vi "RRTAlgorithm2.vi"(0 "Dest x,y":dbl[](array[numeric]), 1 "Robot":T1={"id"=0, "function"=enum."Attacker", "x"=0.0, "y"=0.0, "orientation"=0.0, "v_tangent"=0.0, "v_normal"=0.0, "v_ang"=0.0, "kick_x"=0.0, "kick_z"=0.0, "dribble"=FALSE, "Timestamp"=timestamp(0 s since 1904-01-01), "estimatives"={"est_v_tangent"=0.0, "est_v_normal"=0.0, "est_vx"=0.0, "est_vy"=0.0, "Pos Robot Est"=[]}, "dest_x_kick"=0.0, "dest_y_kick"=0.0, "Gap Coord"=[], "States"=enum."Pass", "Path "=[], "Path  Smooth"=[], "Dest"=[], "vx_desired"=0.0, "vy_desired"=0.0, "slowBehavior"=FALSE, "VSSStates"=enum."Pass"}, 2 "WayPointProb":dbl, 3 "Path in \n(Smooth do Feedback Node)":dbl[][](array[numeric]), 4 "Step":dbl, 5 "GoalProb":dbl, 6 "Simple Path":dbl[][](array[numeric]), 7 "Ball":T7, 8 "Initial Pos x,y":dbl[](array[numeric]), 9 "our_robots":T1[](array[typedef]), 10 "Initial Pos 1,x,y,0":dbl[](array[numeric]), 11 "enemy_robots":T1[](array[typedef]), 12 "ignoreBall?":bool, 13 "Field Geomtery":u32[](array[numeric]), 19 "buffer":dbl[](array[numeric])) -> (16 "Path":dbl[][](array[numeric]))   [LabVIEW 2020]
uses:
  Vision_class/Old vision/SSL Detection Frame Simple Estimator Cameras VelCmd Folder/Core/AI Ball.ctl
  Vision_class/Old vision/Controls/AI Robot.ctl
  Vision_class/Old vision/Controls/Functions Enum.ctl
  Vision_class/Old vision/Controls/AttackerStates.ctl
  Vision_class/Old vision/Controls/PathDests.ctl
  Vision_class/Old vision/Controls/PathDest.ctl
  Navigation/VSSNavigation/VSSAttackerStates.ctl
  <vilib>/Analysis/_algsub.llb/Real Vector Norm.vi
  <vilib>/Analysis/coordinate.llb/2D Cartesian Coordinate Rotation (Scalar).vi
  <vilib>/Analysis/NI_AALPro.lvlib
panel:
  out "useSimplePath":i32
  out "pathsize":i32
  out "debug":sgl
  out "newTree":dbl[](array[numeric])
  in  "threshold":dbl=80.0
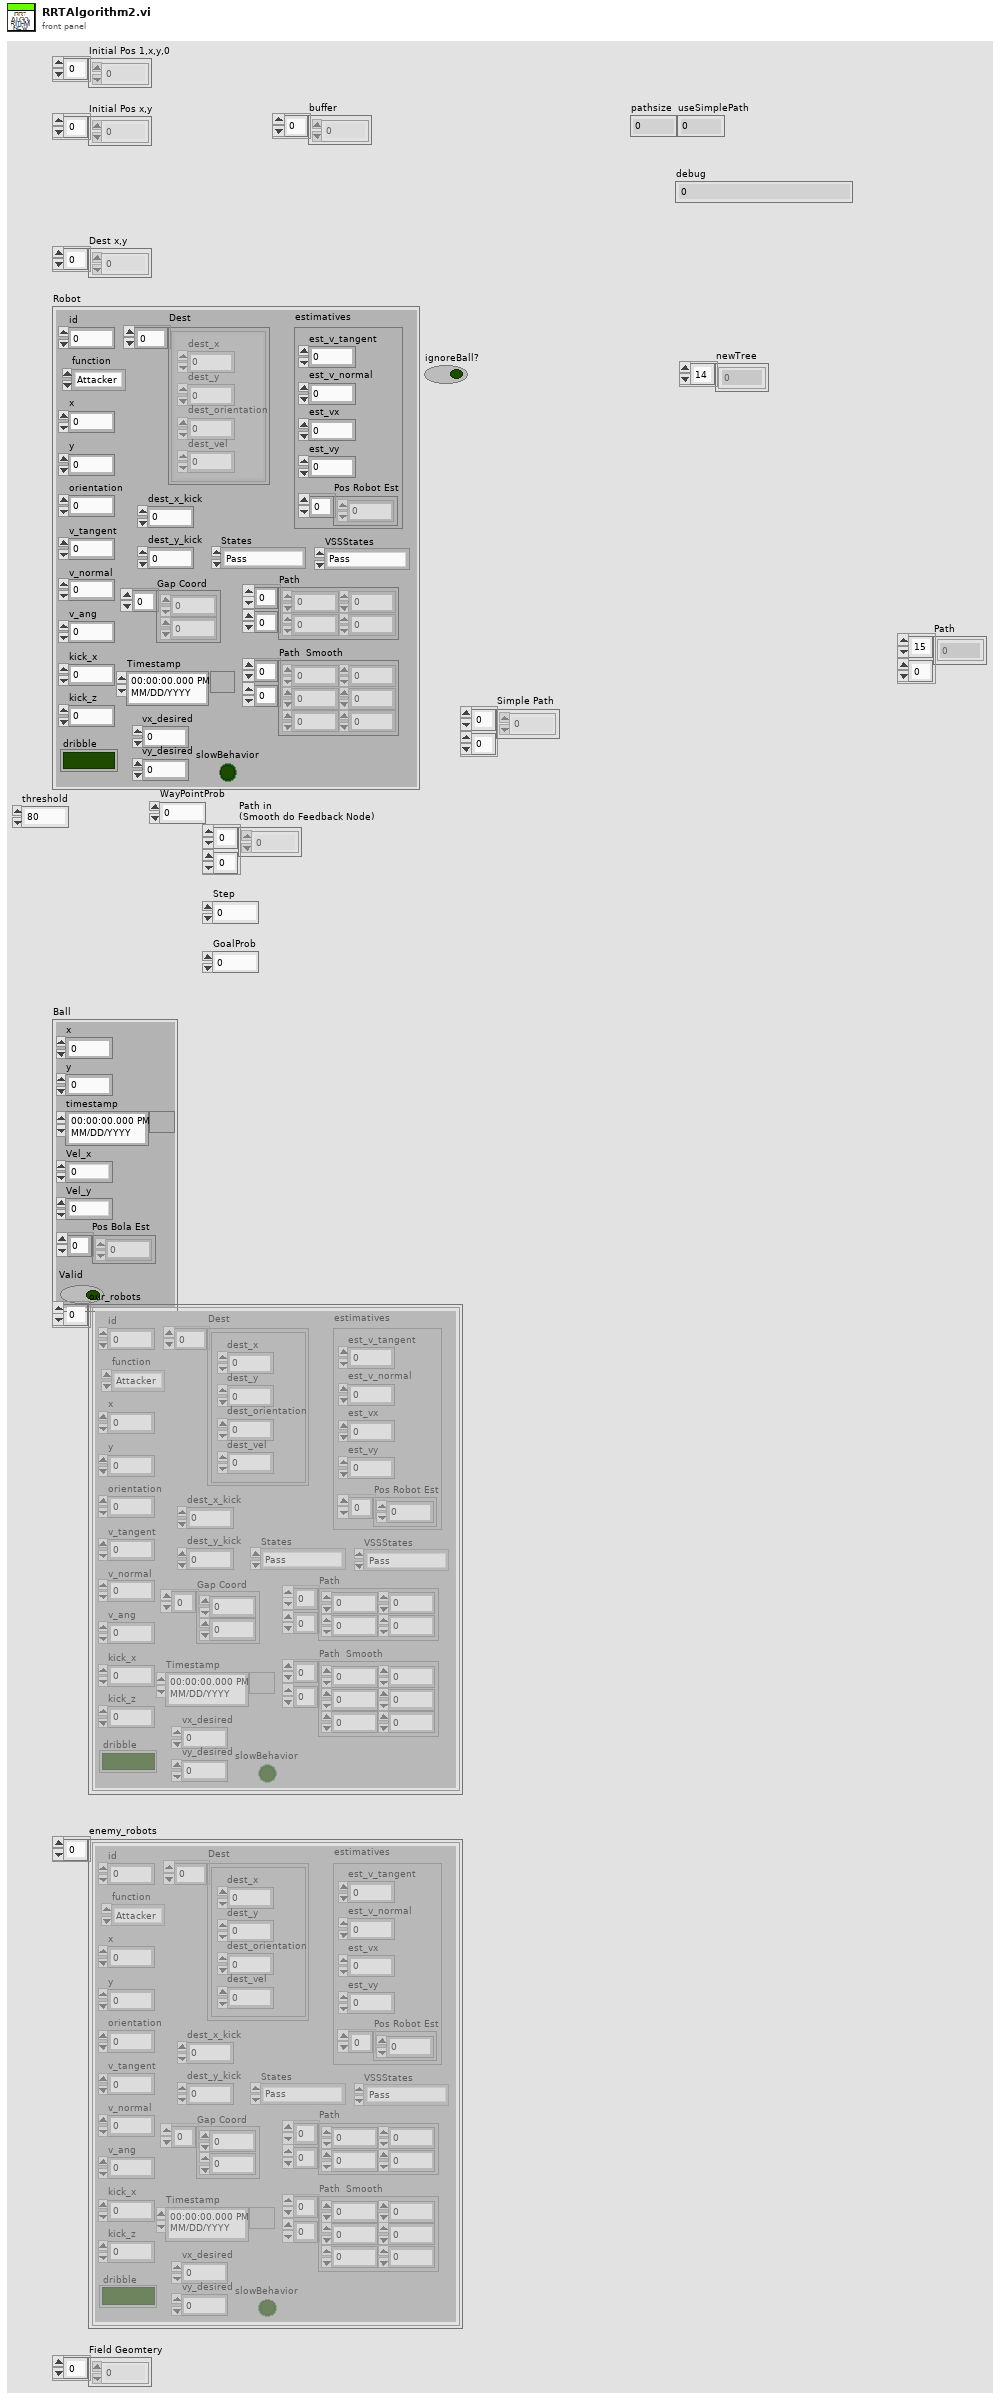
[diagram p1: front panel]
types:
  T1 = typedef "AI Robot.ctl" = cluster{"id":u32, "function":T2, "x":dbl, "y":dbl, "orientation":dbl, "v_tangent":dbl, "v_normal":dbl, "v_ang":dbl, "kick_x":dbl, "kick_z":dbl, "dribble":bool, "Timestamp":timestamp, "estimatives":cluster{"est_v_tangent":dbl, "est_v_normal":dbl, "est_vx":dbl, "est_vy":dbl, "Pos Robot Est":dbl[]}, "dest_x_kick":dbl, "dest_y_kick":dbl, "Gap Coord":dbl[], "States":T3, "Path ":dbl[][], "Path  Smooth":dbl[][], "Dest":T4, "vx_desired":dbl, "vy_desired":dbl, "slowBehavior":bool, "VSSStates":T6}
  T2 = typedef "Functions Enum.ctl" = enum16{"2nd Striker", "Attacker", "Goalie", "Defender", "Striker", "Goto 0", "Dummy", "Kicker", "ZigZag 0", "ZigZag 1", "ZigZag 2", "ZigZag 3", "ZigZag 4", "ZigZag 5", "ZigZag 6", "ZigZag 7", "ZigZag 8", ""}
  T3 = typedef "AttackerStates.ctl" = enum16{"Pass", "GoToTangent", "BallGetting", "GoToKick", ""}
  T4 = typedef "PathDests.ctl" = T5[]
  T5 = typedef "PathDest.ctl" = cluster{"dest_x":dbl, "dest_y":dbl, "dest_orientation":dbl, "dest_vel":dbl}
  T6 = typedef "VSSAttackerStates.ctl" = enum16{"Pass", "GoToTangent", "BallGetting", "GoToKick", "Rotate anti-clockwise", "Rotate Clockwise", ""}
  T7 = typedef "AI Ball.ctl" = cluster{"x":dbl, "y":dbl, "timestamp":timestamp, "Vel_x":dbl, "Vel_y":dbl, "Pos Bola Est":dbl[], "Valid":bool}
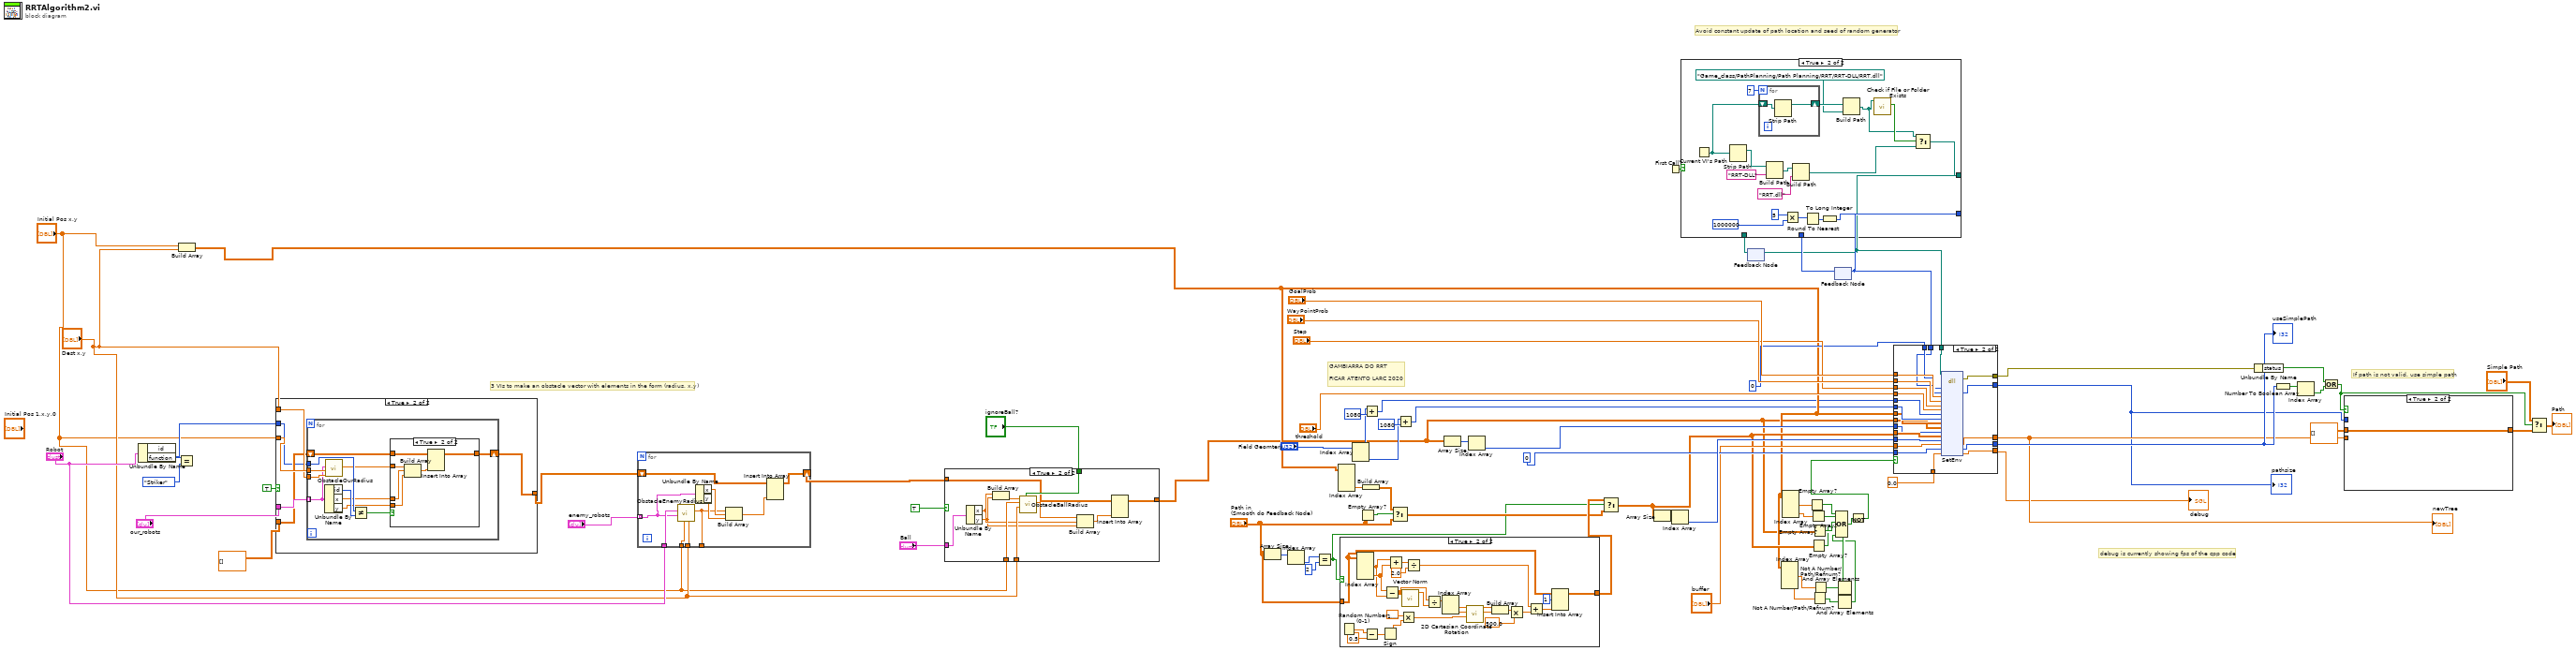
[diagram p0: block diagram]
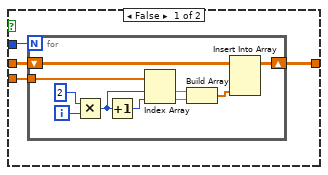
[diagram p4: hidden frame]
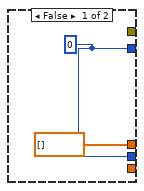
[diagram p5: hidden frame]
diagram:
  # "GAMBIARRA DO RRT\n\nFICAR ATENTO LARC 2020"
  # "debug is currently showing fps of the cpp code"
  # "If path is not valid, use simple path"
  # "3 VIs to make an obstacle vector with elements in the form (radius, x,y)"
  # "Avoid constant update of path location and seed of random generator"
  n1 = Unbundle By Name("Robot") -> ("id"=w66:u32, "function"=w70:T2)
  n2 = Equal?(x=w70, y=Functions_Enum."Striker" ("function")) -> ()  [unwired: 1 out]
  n3 = Build Array("Initial Pos x,y", "Dest x,y") -> (w9:dbl[][])
  n4 = case shown="True" TRUE {
    tunnel: "our_robots" -> [_ w86]
    tunnel: "Initial Pos x,y" -> [_ w85]
    tunnel: "Dest x,y" -> [_ w84]
    tunnel: dbl[][] [] ("appended array") -> [w80 w83]
    tunnel: [w80 w81] -> w63
    tunnel: w66 -> [_ w82]
    frame False {
    }
    frame True {
      n5 = for {
        tunnel: w86 -> [w95] mode=indexing
        tunnel: w85 -> [w97]
        tunnel: w84 -> [w96]
        shift-right: [w87] -> w81
        shift-left: w83 -> [w91]
        tunnel: w82 -> [w93]
        n6 = Unbundle By Name(w95) -> ("id"=w94:u32, "x"=w89:dbl, "y"=w88:dbl)
        n7 = call "ObstacleOurRadius.vi"("Goal"=w96, "Initial State"=w97, "other robot"=w95) -> ("obstacle enemy radius"=w90:dbl)  [unwired: 8 in]
        n8 = Not Equal?(x=w93, y=w94) -> (x != y?=w92:bool)
        n9 = case shown="True" w92 {
          tunnel: w91 -> [w98 w101]
          tunnel: [w98 w99] -> w87
          tunnel: w90 -> [_ w104]
          tunnel: w89 -> [_ w103]
          tunnel: w88 -> [_ w102]
          frame False {
          }
          frame True {
            n10 = Build Array(w104, w103, w102) -> (w100:dbl[])
            n11 = Insert Into Array(array=w101, new element=w100) -> (w99:dbl[][])  [unwired: 2 in]
          }
        }
      }
    }
  }
  n12 = for {
    tunnel: "enemy_robots" -> [w111] mode=indexing
    tunnel: "Initial Pos x,y" -> [w114]
    tunnel: "Dest x,y" -> [w113]
    tunnel: "Robot" -> [w112]
    shift-right: [w106] -> w59
    shift-left: w63 -> [w108]
    tunnel: [w105] -> _
    n13 = call "ObstacleEnemyRadius.vi"("Goal"=w113, "Initial State"=w114, "Robot enemy"=w111, "Robot in"=w112) -> ("obstacle enemy radius"=w105:dbl)  [unwired: 7 in]
    n14 = Unbundle By Name(w111) -> ("x"=w110:dbl, "y"=w109:dbl)
    n15 = Build Array(w105, w110, w109) -> (w107:dbl[])
    n16 = Insert Into Array(array=w108, new element=w107) -> (w106:dbl[][])  [unwired: 2 in]
  }
  n17 = case shown="True" TRUE {
    tunnel: "Ball" -> [_ w126]
    tunnel: "Initial Pos x,y" -> [_ w124]
    tunnel: "Dest x,y" -> [_ w123]
    tunnel: "ignoreBall?" -> [_ w122]
    tunnel: w59 -> [w115 w121]
    tunnel: [w115 w120] -> w1
    frame False {
    }
    frame True {
      n18 = Unbundle By Name(w126) -> ("x"=w118:dbl, "y"=w117:dbl)
      n19 = Build Array(w118, w117) -> (w125:dbl[])
      n20 = call "ObstacleBallRadius.vi"("ignoreBall?"=w122, "Goal"=w123, "Initial State"=w124, "ball"=w125) -> ("obstacle enemy radius"=w119:dbl)  [unwired: 7 in]
      n21 = Build Array(w119, w118, w117) -> (w116:dbl[])
      n22 = Insert Into Array(array=w121, new element=w116) -> (w120:dbl[][])  [unwired: 2 in]
    }
  }
  n23 = Array Size(array="Path in \n(Smooth do Feedback Node)") -> (size(s)=w37:i32[])
  n24 = Index Array(array=w37) -> (element=w36:i32)  [unwired: 1 in]
  n25 = Equal?(x=w36, y=2) -> (x = y?=w31:bool)
  n26 = Index Array(array=w9) -> (element #2=w54:dbl[])  [unwired: 4 in, 1 out]
  n27 = case shown="True" w31 {
    tunnel: "Path in \n(Smooth do Feedback Node)" -> [w127 w134]
    tunnel: [w127 w131] -> w33
    frame False {
    }
    frame True {
      n28 = Random Number (0-1)() -> (number: 0 to 1=w128:dbl)
      n29 = Index Array(array=w134) -> (element #1=w149:dbl[], element #2=w150:dbl[])  [unwired: 4 in]
      n30 = Subtract(x=w128, y=0.5) -> (x-y=w130:dbl)
      n31 = Sign(1:w130) -> (0:w145:dbl)
      n32 = Subtract(x=w150, y=w149) -> (x-y=w147:dbl[])
      n33 = Add(x=w149, y=w150) -> (x+y=w152:dbl[])
      n34 = Multiply(x=1.5707963267948966, y=w145) -> (x*y=w144:dbl)
      n35 = call-poly <vilib>:"Vector Norm.vi"("Input Vector"=w147) -> ("norm"=w148:dbl)  [unwired: 9 in, 1 out]
      n36 = Divide(x=w152, y=2.0) -> (x/y=w135:dbl[])
      n37 = Divide(x=w147, y=w148) -> (x/y=w143:dbl[])
      n38 = Index Array(array=w143) -> (element #1=w142:dbl, element #2=w141:dbl)  [unwired: 2 in]
      n39 = call-poly <vilib>:"2D Cartesian Coordinate Rotation.vi"("theta"=w144, "y"=w141, "x"=w142) -> ("y out"=w139:dbl, "x out"=w140:dbl)  [unwired: 6 in, 1 out]
      n40 = Build Array(w140, w139) -> (w137:dbl[])
      n41 = Multiply(x=w137, y=500.0) -> (x*y=w136:dbl[])
      n42 = Add(x=w135, y=w136) -> (x+y=w132:dbl[])
      n43 = Insert Into Array(array=w134, index (row)=1, new element=w132) -> (w131:dbl[][])  [unwired: 1 in]
    }
  }
  n44 = Index Array(array="Field Geomtery") -> (element #1=w4:u32, element #2=w7:u32)  [unwired: 2 in]
  n45 = Empty Array?(array="Path in \n(Smooth do Feedback Node)") -> (empty?=w55:bool)
  n46 = Build Array(w54) -> (w47:dbl[][])
  n47 = Add(x=w4, y=u32 1080) -> (x+y=w3:u32)
  n48 = Select(t=w47, s=w55, f="Path in \n(Smooth do Feedback Node)") -> (s? t:f=w32:dbl[][])
  n49 = Add(x=w7, y=u32 1080) -> (x+y=w6:u32)
  n50 = Array Size(array=w1) -> (size(s)=w57:i32[])
  n51 = Index Array(array=w57) -> (element=w73:i32)  [unwired: 1 in]
  n52 = Select(t=w33, s=w31, f=w32) -> (s? t:f=w27:dbl[][])
  n53 = Array Size(array=w27) -> (size(s)=w56:i32[])
  n54 = First Call?() -> (First Call?: T/F=w44:bool)
  n55 = Index Array(array=w56) -> (element=w75:i32)  [unwired: 1 in]
  n56 = feedback #1() -> (w43:path)  [unwired: 1 in]
  n57 = Index Array(array=w9) -> (element #1=w16:dbl[], element #2=w15:dbl[])  [unwired: 4 in]
  n58 = Index Array(array=w9) -> (element #1=w29:dbl[], element #2=w28:dbl[])  [unwired: 4 in]
  n59 = Empty Array?(array=w29) -> (empty?=w18:bool)
  n60 = Empty Array?(array=w28) -> (empty?=w17:bool)
  n61 = Empty Array?(array=w27) -> (empty?=w25:bool)
  n62 = Empty Array?(array=w1) -> (empty?=w26:bool)
  n63 = Not A Number/Path/Refnum?(number/path/refnum=w15) -> (NaN/Path/Refnum?=w13:bool[])
  n64 = Not A Number/Path/Refnum?(number/path/refnum=w16) -> (NaN/Path/Refnum?=w14:bool[])
  n65 = feedback #2() -> (w41:i32)  [unwired: 1 in]
  n66 = case shown="True" w44 {
    tunnel: [w154 w158] -> w39
    tunnel: w43 -> [w154 _]
    tunnel: [w153 w166] -> w40
    tunnel: w41 -> [w153 _]
    frame False {
    }
    frame True {
      n67 = Current VI's Path() -> (path=w162:path)
      n68 = Strip Path(path=w162) -> (stripped path=w171:path)  [unwired: 1 out]
      n69 = for {
        N: 7 -> [_]
        shift-right: [w172] -> w160
        shift-left: w162 -> [w173]
        n70 = Strip Path(path=w173) -> (stripped path=w172:path)  [unwired: 1 out]
      }
      n71 = Build Path(base path=w171, name or relative path="RRT-DLL") -> (appended path=w164:path)
      n72 = Multiply(x=5, y=1000000) -> (x*y=w168:i32)
      n73 = Build Path(base path=w164, name or relative path="RRT.dll") -> (appended path=w155:path)
      n74 = Round To Nearest(number=w168) -> (nearest integer value=w167:i32)
      n75 = To Long Integer(number=w167) -> (32bit integer=w166:i32)
      n76 = Build Path(base path=w160, name or relative path=path "Game_class/PathPlanning/Path Planning/RRT/RRT-DLL/RRT.dll") -> (appended path=w156:path)
      n77 = call <vilib>:"Check if File or Folder Exists.vi"("path"=w156) -> ("file or folder exists?"=w157:bool)  [unwired: 8 in, 2 out]
      n78 = Select(t=w156, s=w157, f=w155) -> (s? t:f=w158:path)
    }
  }
  n79 = feedback-in #1(w39) -> ()
  n80 = feedback-in #2(w40) -> ()
  n81 = And Array Elements(Boolean array=w14) -> (logical AND=w12:bool)
  n82 = And Array Elements(Boolean array=w13) -> (logical AND=w11:bool)
  n83 = Compound Arithmetic op=OR(w18, w17, w26, w25, w12, w11) -> (w24:bool)
  n84 = Not(x=w24) -> (.not. x?=w10:bool)
  n85 = case shown="True" w10 {
    tunnel: "GoalProb" -> [_ w197]
    tunnel: "WayPointProb" -> [_ w196]
    tunnel: "Step" -> [_ w195]
    tunnel: "threshold" -> [_ w194]
    tunnel: w3 -> [_ w193]
    tunnel: w6 -> [_ w192]
    tunnel: w9 -> [_ w191]
    tunnel: w1 -> [_ w190]
    tunnel: w27 -> [_ w189]
    tunnel: w75 -> [_ w188]
    tunnel: 0 -> [_ w187]
    tunnel: "buffer" -> [_ w186]
    tunnel: [dbl[] [] ("newTree") w185] -> w71
    tunnel: [w174 w184] -> w72
    tunnel: [w174 w177] -> w38
    tunnel: w73 -> [_ w183]
    tunnel: sgl 0.0 ("debug") -> [_ w181]
    tunnel: 0 -> [_ w182]
    tunnel: [_ w180] -> w42
    tunnel: w40 -> [_ w179]
    tunnel: w39 -> [_ w178]
    tunnel: [_ w176] -> w23
    frame False {
      w174 = 0 ("pathsize")
    }
    frame True {
      n86 = dll-call lib="C:/Users/anton/source/repos/RRT/x64/Release/RRT.dll" fn="SetEnv"(path in=w178, "seed"=w179, "pathsize"=w182, "probGoal"=w197, "probWaypoint"=w196, "step"=w195, "threshold"=w194, "field_length"=w193, "field_width"=w192, "Start/End"=w191, "obsList"=w190, "obsLen"=w183, "lastTree"=w189, "lastTreeLen"=w188, "newTree"=w186, "useSimplePath"=w187, "debug"=w181) -> (error out=w176:errorcluster, "pathsize"=w177:i32, "newTree"=w185:sgl[], "useSimplePath"=w184:i8, "debug"=w180:sgl)  [unwired: 15 in, 1 out]
    }
  }
  "newTree" <- w71
  "debug" <- w42
  "pathsize" <- w38
  "useSimplePath" <- w72
  n87 = Unbundle By Name(w23) -> ("status"=w21:bool)
  n88 = Number To Boolean Array(number=w72) -> (Boolean array=w50:bool[])
  n89 = Index Array(array=w50) -> (element=w22:bool)  [unwired: 1 in]
  n90 = Or(x=w21, y=w22) -> (x .or. y?=w20:bool)
  n91 = case shown="True" w20 {
    tunnel: w71 -> [w201 _]
    tunnel: dbl[][] [] ("s? t:f") -> [w200 w212]
    tunnel: w38 -> [w199 _]
    tunnel: [w198 w212] -> w51
    frame False {
      n92 = for {
        N: w199 -> [_]
        tunnel: w201 -> [w209]
        shift-right: [w202] -> w198
        shift-left: w200 -> [w204]
        i -> [w211]
        n93 = Multiply(x=2, y=w211) -> (x*y=w207:i32)
        n94 = Increment(x=w207) -> (x+1=w208:i32)
        n95 = Index Array(array=w209, index #1=w207, index #2=w208) -> (element #1=w206:dbl, element #2=w205:dbl)
        n96 = Build Array(w206, w205) -> (w203:dbl[])
        n97 = Insert Into Array(array=w204, new element=w203) -> (w202:dbl[][])  [unwired: 2 in]
      }
    }
    frame True {
    }
  }
  n98 = Select(t="Simple Path", s=w20, f=w51) -> (s? t:f=→"Path":dbl[][])
